vi "myFreqGen.vi"(4 "f_dens":u32, 6 "dens":dbl, 8 "f_min":u32, 9 "f_max":u32, 11 "N":u32) -> (2 "freqs":i32[](array[numeric]))   [LabVIEW 2024]
doc: "根据基础设置，初步构建扫频频率值freqs数组。"
uses:
  8248d584-2b4c-4841-ba6c-f30ac45cc9bb.vi
panel:
  # "基础设置\n设置无效内容时请祈祷能自动补全。"
  # "频率上限，\n最高1M (Hz)"
  # "频率下限，\n最低1 (Hz)"
  # "期望频点个数，\n最小2"
  # "密度设置（测试功能，建议禁用）\n设置为无效数据来禁用该部分。"
  # "密度常数，\n小于1.0时无效"
  # "密集频率，\n当密度常数<=1.0时无效"
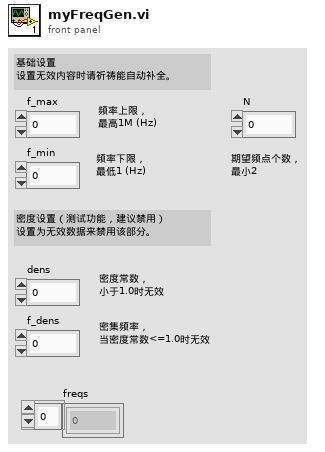
[diagram p1: front panel]
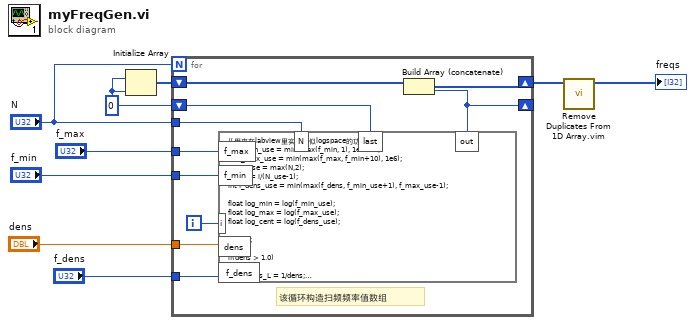
[diagram p0: block diagram]
diagram:
  w7 = 0
  n1 = Initialize Array(w7, w7) -> (w1:i32[])
  n2 = for {
    N: "N" -> [_]
    tunnel: "f_min" -> [w19]
    tunnel: "N" -> [w18]
    tunnel: "f_max" -> [w17]
    shift-right: [w15] -> w8
    shift-left: w1 -> [w14]
    tunnel: "f_dens" -> [w13]
    tunnel: "dens" -> [w12]
    shift-right: [w11] -> _
    shift-left: w7 -> [w10]
    i -> [w16]
    # "该循环构造扫频频率值数组"
    n3 = formula code="// 用来在labview里实现类似logspace的功能\nint f_min_use = min(max(f_min, 1), 1e6-10);\nint f_max_use = min(max(f_max, f_min+10), 1e6);\nint N_use = max(N,2); \nfloat t = i/(N_use-1);\nint f_dens_use = min(max(f_dens, f_min_use+1), f_max_use-1);\n\nfloat log_min = log(f_min_use);\nfloat log_max = log(f_max_use);\nfloat log_cent = log(f_dens_use);\n\nint out;\n\nif(dens > 1.0)\n{\n\tfloat dens_L = 1/dens;\n\tfloat dens_R = dens;\n\n\tfloat log_del_L = pow(log_cent - log_min, 1/dens_L);\n\tfloat log_del_R = pow(log_max - log_cent, 1/dens_R);\n\n\tfloat t_cent = (log_cent-log_min)/(log_max-log_min);\n\tif(t <= t_cent)\n\t{\n\t\tout = pow(10, log_min + pow(t/t_cent * log_del_L, dens_L));\n\t}\n\telse\n\t{\n\t\tout = pow(10, log_cent + pow(((t-t_cent)/(1-t_cent) * log_del_R), dens_R));\n\t}\n}\nelse\n{\n\tout = pow(10, log_min + t*(log_max-log_min));\n}\n\n// 关于分辨率取整\nint delta;\nif(out>=1e5)\n{delta = 1e4;}\nelse if(out>=1e4)\n{delta = 1e3;}\nelse if(out>=1e3)\n{delta = 1e2;}\nelse if(out>=1e2)\n{delta = 1e1;}\nelse\n{delta = 1;}\n\nout = delta * int(out/delta);"("f_min"=w19, "N"=w18, "f_max"=w17, "i"=w16, "dens"=w12, "f_dens"=w13, "last"=w10) -> ("out"=w11:i32)
    n4 = Build Array (concatenate)(w14, w11) -> (w15:i32[])
  }
  n5 = call "Remove Duplicates From 1D Array.vim"("array"=w8) -> ("array with duplicates removed"=→"freqs":i32[])  [unwired: 10 in]
